vi "TORCS_model.vi"(0 "Steer":dbl, 1 "Acceleration":dbl, 2 "RR brake":dbl, 3 "FL brake":dbl, 4 "Brake":dbl, 5 "Gear":dbl, 6 "RL brake":dbl, 7 "FR brake":dbl) -> (8 "speed X":dbl, 11 "Spin Vel 1":dbl, 12 "speed Y":dbl, 14 "Enginr RPM":dbl, 15 "Spin Vel 2":dbl, 16 "speed Z":dbl, 17 "Spin Vel 3":dbl, 20 "Slip ratio":dbl, 21 "Slip Side 1":dbl, 24 "Slip Side 2":dbl, 27 "Spin Vel 4":dbl)   [LabVIEW 2012]
uses:
  DataToSend.ctl
panel:
  out "Slip accel 2":dbl
  in  "stop 2":bool
  in  "Send":dbl
  out "Slip accel 4":dbl
  out "Slip Side 4":dbl
  out "Slip accel 3":dbl
  out "Slip side 3":dbl
  out "Slip accel 1":dbl
  out "acc Z":dbl
  out "acc Y":dbl
  out "acc X":dbl
  out "posZ":dbl
  out "posY":dbl
  out "posX":dbl
  out "Fuel Remain":dbl
  out "Fuel cons.":dbl
  out "Data to read  2":T1
  out "Data in Array":dbl[](array[numeric])
  out "error code":i32
  in  "stop":bool
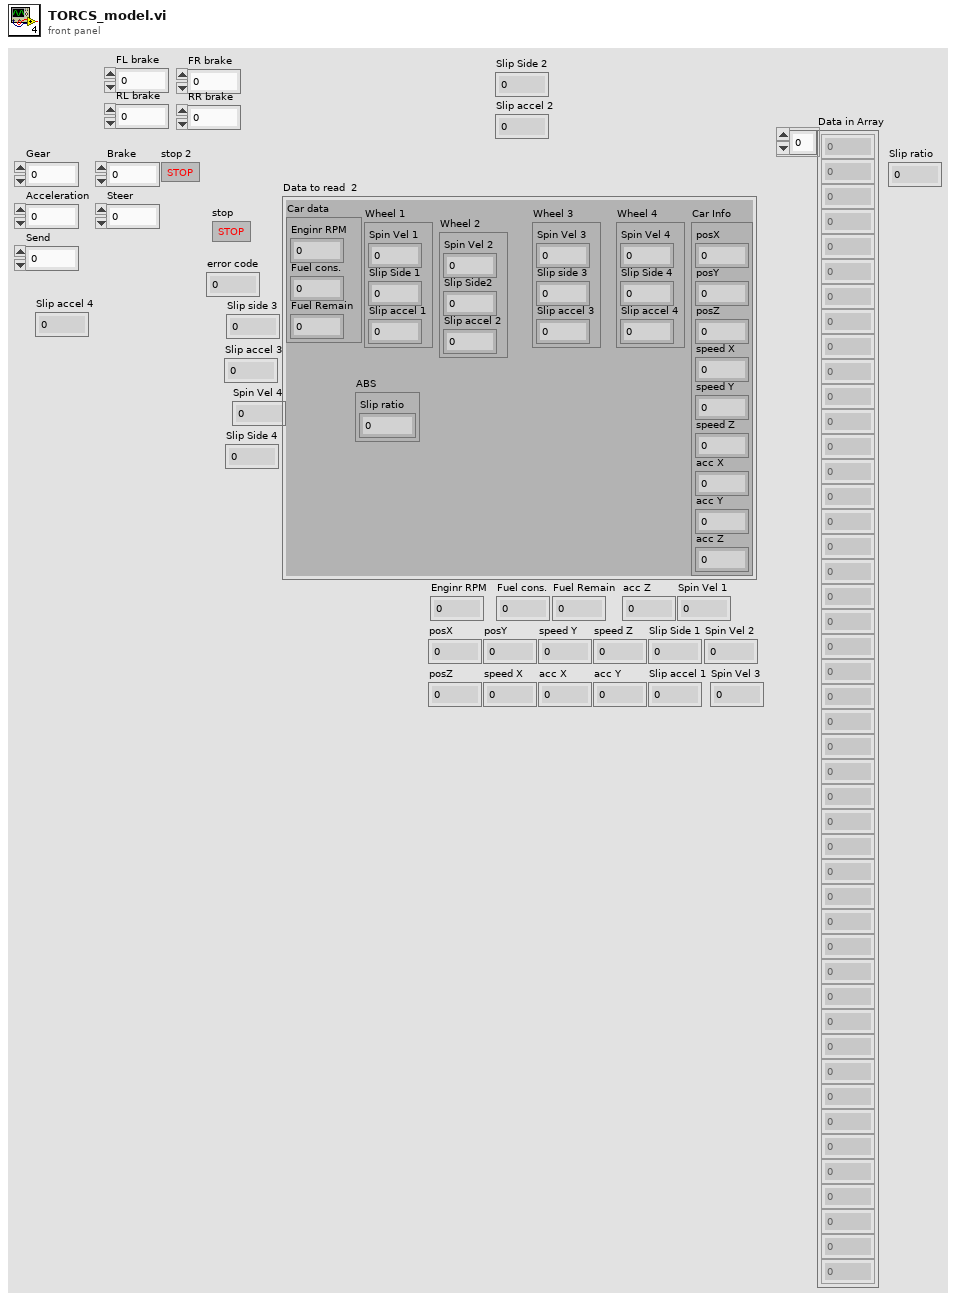
[diagram p1: front panel]
types:
  T1 = cluster{"Car data ":cluster{"Enginr RPM":dbl, "Fuel cons.":dbl, "Fuel Remain":dbl}, "Wheel 1":cluster{"Spin Vel 1":dbl, "Slip Side 1":dbl, "Slip accel 1":dbl}, "Wheel 2":cluster{"Spin Vel 2":dbl, "Slip Side2":dbl, "Slip accel 2":dbl}, "Wheel 3":cluster{"Spin Vel 3":dbl, "Slip side 3":dbl, "Slip accel 3":dbl}, "Wheel 4":cluster{"Spin Vel 4":dbl, "Slip Side 4":dbl, "Slip accel 4":dbl}, "Car Info":cluster{"posX":dbl, "posY":dbl, "posZ":dbl, "speed X":dbl, "speed Y":dbl, "speed Z":dbl, "acc X":dbl, "acc Y":dbl, "acc Z":dbl}, "ABS":cluster{"Slip ratio":dbl}}
  T2 = cluster{"Remote Host Port":u16, "Remote Host IP":string, "write_ID":enum32{"0", "1", "2", "3", "4"}}
  T3 = typedef "DataToSend.ctl" = cluster{"Gear":dbl, "Acceleration":dbl, "Brake":dbl, "Steer":dbl, "Send":dbl, "FR brake":dbl, "FL brake":dbl, " RR brake":dbl, " RL brake":dbl}
  T4 = cluster{"Enginr RPM":dbl, "Fuel cons.":dbl, "Fuel Remain":dbl}
  T5 = cluster{"posX":dbl, "posY":dbl, "posZ":dbl, "speed X":dbl, "speed Y":dbl, "speed Z":dbl, "acc X":dbl, "acc Y":dbl, "acc Z":dbl}
  T6 = cluster{"Spin Vel 1":dbl, "Slip Side 1":dbl, "Slip accel 1":dbl}
  T7 = cluster{"Spin Vel 2":dbl, "Slip Side2":dbl, "Slip accel 2":dbl}
  T8 = cluster{"Spin Vel 3":dbl, "Slip side 3":dbl, "Slip accel 3":dbl}
  T9 = cluster{"Spin Vel 4":dbl, "Slip Side 4":dbl, "Slip accel 4":dbl}
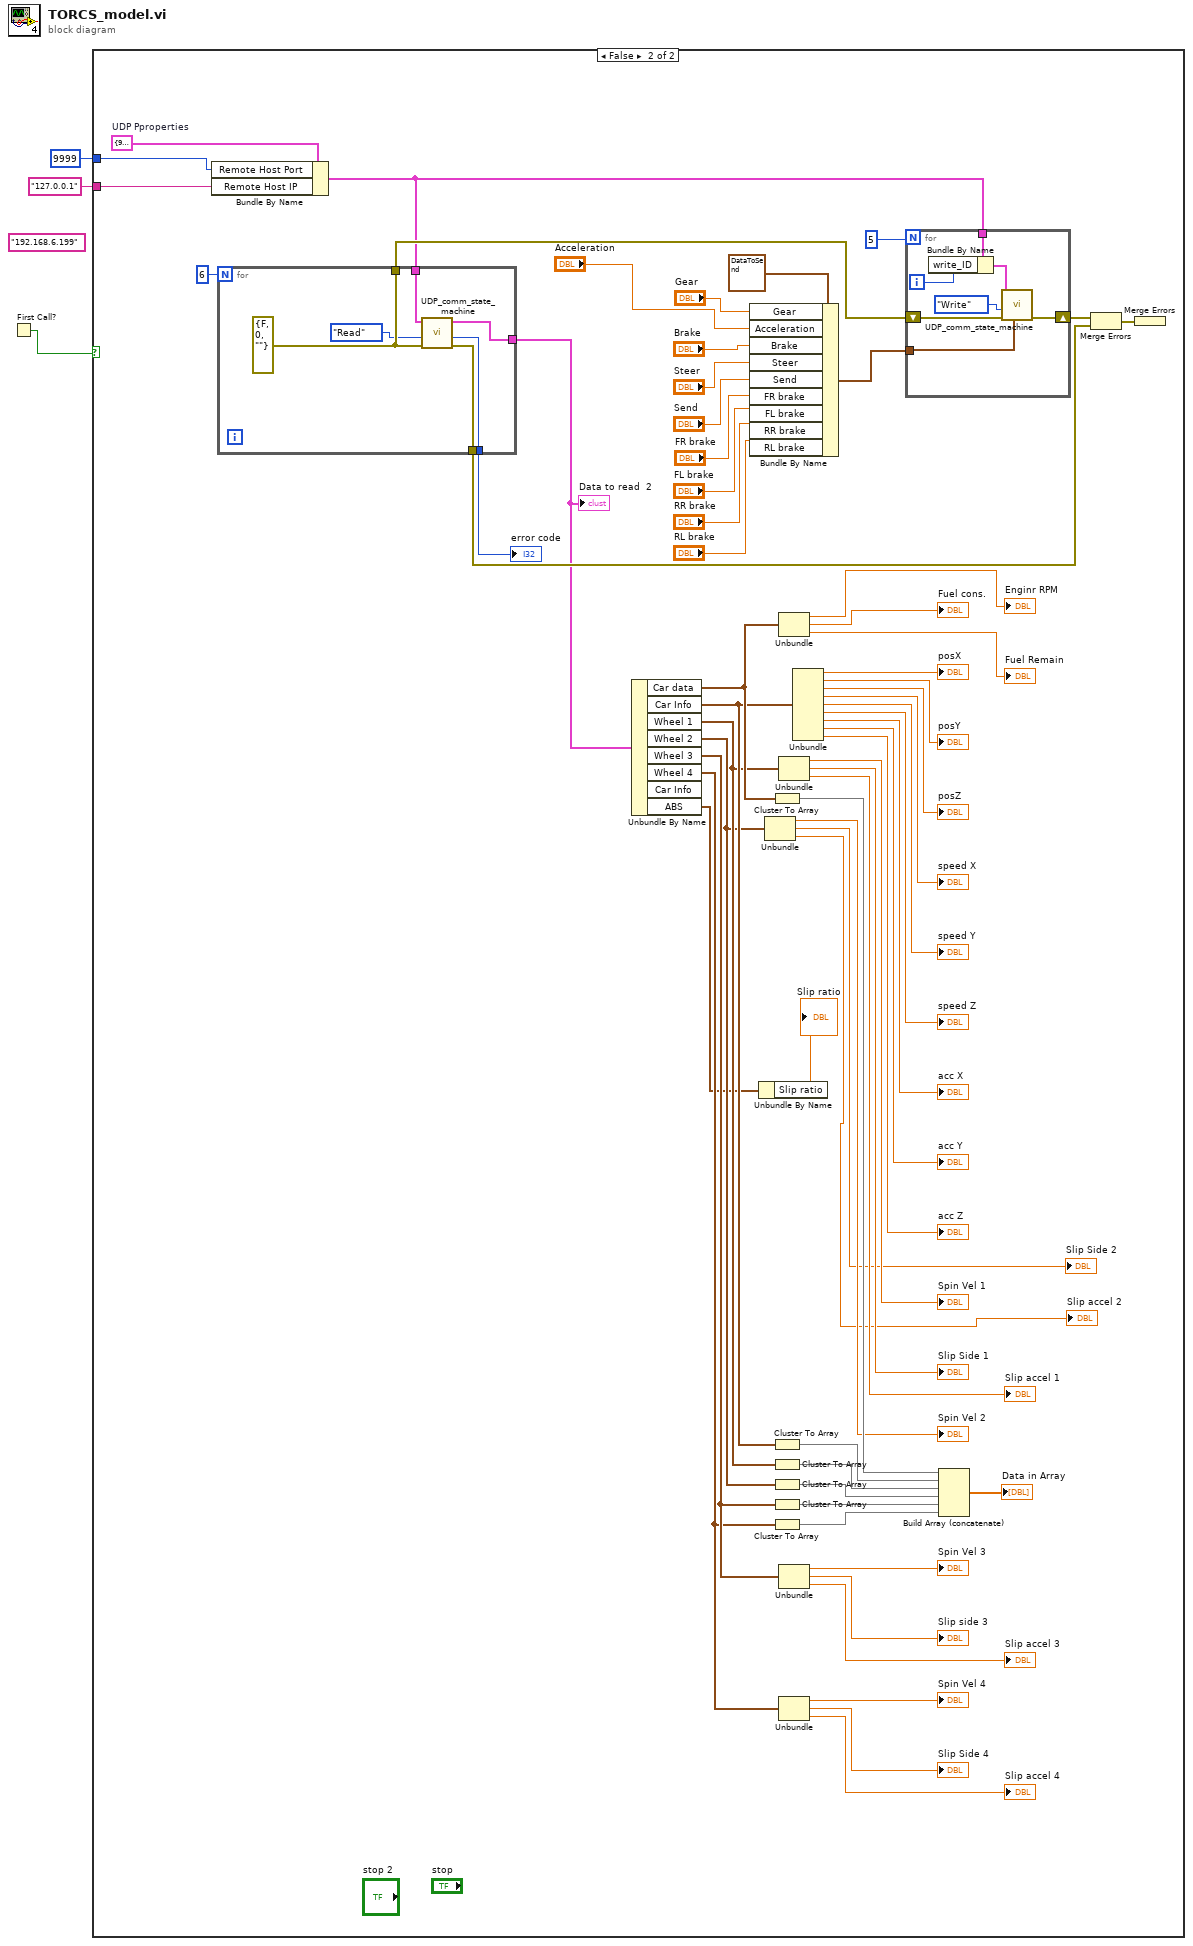
[diagram p0: block diagram]
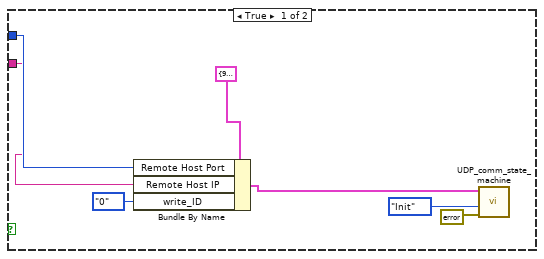
[diagram p2: hidden frame]
diagram:
  (unwired) "192.168.6.199" ("Remote Host IP")
  n1 = First Call?() -> (First Call?: T/F=w1:bool)
  n2 = case shown="False" w1 {
    tunnel: "127.0.0.1" ("Remote Host IP") -> [w6 w72]
    tunnel: u16 9999 ("Remote Host Port") -> [w7 w71]
    frame True {
      n3 = Bundle By Name(cluster=T2 {"Remote Host Port"=9999, "Remote Host IP"="192.168.6.190", "write_ID"=enum."0"} ("UDP Pproperties"), "Remote Host Port"=w7, "Remote Host IP"=w6, "write_ID"=enum32{"0", "1", "2", "3", "4"}."0") -> (w4:T2)
      n4 = call "UDP_comm_state_machine.vi"("error in (no error)"=errorcluster {"status"=FALSE, "code"=0, "source"=""}, "UDP State"=enum16{"Init", "Write", "Read", "Close"}."Init", "UDP Pproperties"=w4) -> ()  [unwired: 6 in, 3 out]
    }
    frame False {
      w69 = T2 {"Remote Host Port"=9999, "Remote Host IP"="10.92.1.34", "write_ID"=enum."0"}  # UDP Pproperties
      n5 = Bundle By Name(cluster=w69, "Remote Host Port"=w71, "Remote Host IP"=w72) -> (w18:T2)
      n6 = for {
        N: 6 -> [_]
        tunnel: [w78] -> w68
        tunnel: [w76] -> w67
        tunnel: [w75] -> w58
        tunnel: w18 -> [w74]
        tunnel: [w73] -> w17
        w78 = errorcluster {"status"=FALSE, "code"=0, "source"=""} ("error IO")
        n7 = call "UDP_comm_state_machine.vi"("error in (no error)"=w78, "UDP State"=enum16{"Init", "Write", "Read", "Close"}."Read", "UDP Pproperties"=w74) -> ("error out"=w75:errorcluster, "error code"=w76:i32, "Data to read OUT"=w73:T1)  [unwired: 6 in]
      }
      "error code" <- w67
      "Data to read  2" <- w17
      n8 = Unbundle By Name(w17) -> ("Car data"=w57:T4, "Car Info"=w56:T5, "Wheel 1"=w55:T6, "Wheel 2"=w54:T7, "Wheel 3"=w53:T8, "Wheel 4"=w52:T9, "ABS"=w23:cluster{"Slip ratio":dbl})  [unwired: 1 out]
      n9 = Bundle By Name(cluster=T3 {"Gear"=0.0, "Acceleration"=0.0, "Brake"=0.0, "Steer"=0.0, "Send"=0.0, "FR brake"=0.0, "FL brake"=0.0, " RR brake"=0.0, " RL brake"=0.0} ("Data to send"), "Gear"="Gear", "Acceleration"="Acceleration", "Brake"="Brake", "Steer"="Steer", "Send"="Send", "FR brake"="FR brake", "FL brake"="FL brake", "RR brake"="RR brake", "RL brake"="RL brake") -> (w29:T3)
      n10 = Unbundle By Name(w23) -> ("Slip ratio"=→"Slip ratio":dbl)
      n11 = Unbundle(w54) -> ("Spin Vel 2"=→"Spin Vel 2":dbl, "Slip Side2"=→"Slip Side 2":dbl, "Slip accel 2"=→"Slip accel 2":dbl)
      n12 = Cluster To Array(cluster=w57) -> (array=w66:dbl[])
      n13 = Cluster To Array(cluster=w56) -> (array=w65:dbl[])
      n14 = Cluster To Array(cluster=w55) -> (array=w64:dbl[])
      n15 = Cluster To Array(cluster=w54) -> (array=w63:dbl[])
      n16 = Cluster To Array(cluster=w53) -> (array=w62:dbl[])
      n17 = Cluster To Array(cluster=w52) -> (array=w61:dbl[])
      n18 = Unbundle(w57) -> ("Enginr RPM"=→"Enginr RPM":dbl, "Fuel cons."=→"Fuel cons.":dbl, "Fuel Remain"=→"Fuel Remain":dbl)
      n19 = Unbundle(w55) -> ("Spin Vel 1"=→"Spin Vel 1":dbl, "Slip Side 1"=→"Slip Side 1":dbl, "Slip accel 1"=→"Slip accel 1":dbl)
      n20 = Unbundle(w53) -> ("Spin Vel 3"=→"Spin Vel 3":dbl, "Slip side 3"=→"Slip side 3":dbl, "Slip accel 3"=→"Slip accel 3":dbl)
      n21 = Unbundle(w52) -> ("Spin Vel 4"=→"Spin Vel 4":dbl, "Slip Side 4"=→"Slip Side 4":dbl, "Slip accel 4"=→"Slip accel 4":dbl)
      n22 = Unbundle(w56) -> ("posX"=→"posX":dbl, "posY"=→"posY":dbl, "posZ"=→"posZ":dbl, "speed X"=→"speed X":dbl, "speed Y"=→"speed Y":dbl, "speed Z"=→"speed Z":dbl, "acc X"=→"acc X":dbl, "acc Y"=→"acc Y":dbl, "acc Z"=→"acc Z":dbl)
      n23 = for {
        N: 5 -> [_]
        tunnel: w29 -> [w79]
        shift-right: [w83] -> w59
        shift-left: w68 -> [w85]
        tunnel: w18 -> [w82]
        i -> [w80]
        n24 = Bundle By Name(cluster=w82, "write_ID"=w80) -> (w81:T2)
        n25 = call "UDP_comm_state_machine.vi"("Data to send"=w79, "error in (no error)"=w85, "UDP State"=enum16{"Init", "Write", "Read", "Close"}."Write", "UDP Pproperties"=w81) -> ("error out"=w83:errorcluster)  [unwired: 5 in, 2 out]
      }
      n26 = Build Array (concatenate)(w66, w65, w64, w63, w62, w61) -> (→"Data in Array":dbl[])
      n27 = Merge Errors(w59, w58) -> (w70:errorcluster)
      n28 = Merge Errors(w70) -> ()  [unwired: 1 out]
    }
  }
